vi "Choose Elevator Load Position.vi"(6 "Have Totes?":bool, 9 "Have Trashcan?":bool, 10 "Presets":T2, 11 "Command":T1) -> (3 "Elevator Position":dbl)   [LabVIEW 2014]
uses:
  Elevator Presets.ctl
  Elevator Command.ctl
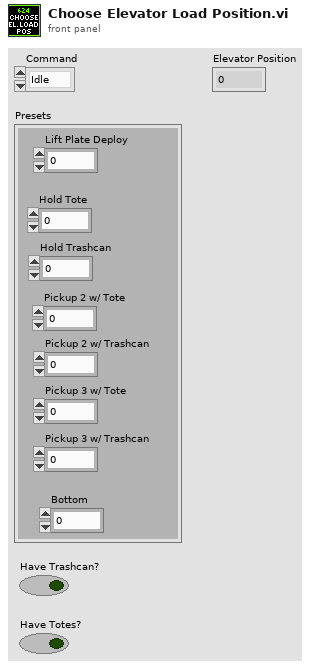
[diagram p1: front panel]
types:
  T1 = typedef "Elevator Command.ctl" = enum16{"Idle", "Load 1", "Load 2", "Load 3", "Drop Stack", "Eject Stack"}
  T2 = typedef "Elevator Presets.ctl" = cluster{"Hold Tote":dbl, "Hold Trashcan":dbl, "Pickup 2 w/ Tote":dbl, "Pickup 2 w/ Trashcan":dbl, "Pickup 3 w/ Tote":dbl, "Pickup 3 w/ Trashcan":dbl, "Lift Plate Deploy":dbl, "Bottom":dbl}
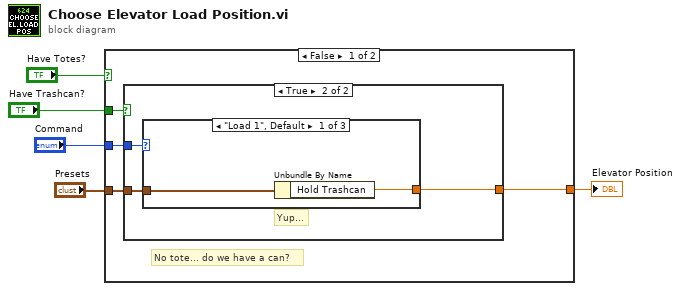
[diagram p0: block diagram]
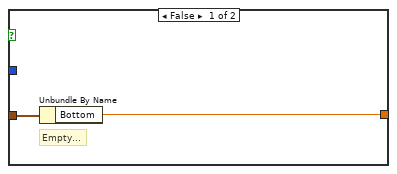
[diagram p2: hidden frame]
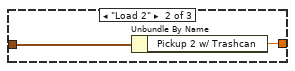
[diagram p3: hidden frame]
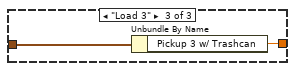
[diagram p4: hidden frame]
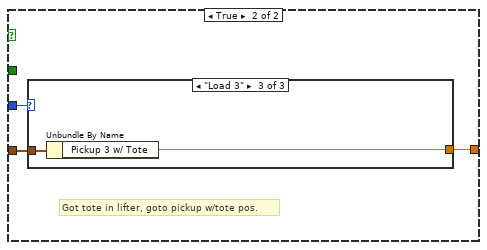
[diagram p5: hidden frame]
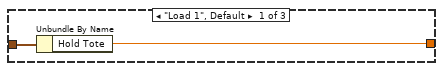
[diagram p6: hidden frame]
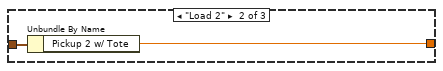
[diagram p7: hidden frame]
diagram:
  n1 = case shown="False" "Have Totes?" {
    tunnel: "Command" -> [w8 w23]
    tunnel: "Presets" -> [w7 w22]
    tunnel: [w6 w21] -> w4
    tunnel: "Have Trashcan?" -> [w9 _]
    frame False {
      # "No tote... do we have a can?"
      n2 = case shown="True" w9 {
        tunnel: w8 -> [_ w14]
        tunnel: w7 -> [w11 w13]
        tunnel: [w10 w12] -> w6
        frame False {
          # "Empty..."
          n3 = Unbundle By Name(w11) -> ("Bottom"=w10:dbl)
        }
        frame True {
          # "Yup..."
          n4 = case shown="\"Load 1\", Default" w14 {
            tunnel: w13 -> [w16 w18 w20]
            tunnel: [w15 w17 w19] -> w12
            frame "Load 1", Default {
              n5 = Unbundle By Name(w16) -> ("Hold Trashcan"=w15:dbl)
            }
            frame "Load 2" {
              n6 = Unbundle By Name(w18) -> ("Pickup 2 w/ Trashcan"=w17:dbl)
            }
            frame "Load 3" {
              n7 = Unbundle By Name(w20) -> ("Pickup 3 w/ Trashcan"=w19:dbl)
            }
          }
        }
      }
    }
    frame True {
      # "Got tote in lifter, goto pickup w/tote pos."
      n8 = case shown="\"Load 3\"" w23 {
        tunnel: w22 -> [w25 w27 w29]
        tunnel: [w24 w26 w28] -> w21
        frame "Load 1", Default {
          n9 = Unbundle By Name(w25) -> ("Hold Tote"=w24:dbl)
        }
        frame "Load 2" {
          n10 = Unbundle By Name(w27) -> ("Pickup 2 w/ Tote"=w26:dbl)
        }
        frame "Load 3" {
          n11 = Unbundle By Name(w29) -> ("Pickup 3 w/ Tote"=w28:dbl)
        }
      }
    }
  }
  "Elevator Position" <- w4
